vi "Generate Header Vectors.vi"(0 "RFFE RegReadExt Command in":refnum<class "RFFE RegReadExt Command.lvclass">, 11 "error in (no error)":errorcluster) -> (4 "RFFE RegReadExt Command out":refnum<class "RFFE RegReadExt Command.lvclass">, 6 "Header Vectors":string[](array[string]), 15 "error out":errorcluster)   [LabVIEW 2018, in "MIPI RFFE API.lvlib" / "RFFE RegReadExt Command.lvclass"]
uses:
  RFFE RegReadExt Command.lvclass
  Extended Command/RFFE Extended Command.lvclass
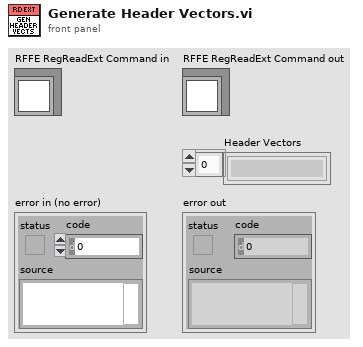
[diagram p1: front panel]
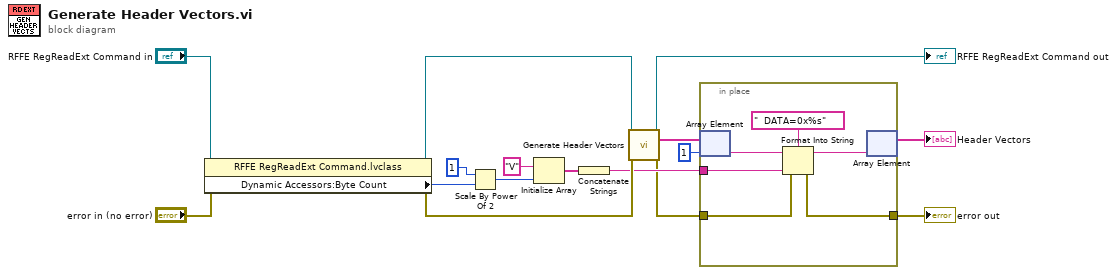
[diagram p0: block diagram]
diagram:
  n1 = property class="RFFE RegReadExt Command.lvclass"(reference="RFFE RegReadExt Command in", error in="error in (no error)") -> (reference out=w14:refnum<class "RFFE RegReadExt Command.lvclass">, error out=w8:errorcluster, "Dynamic Accessors:Byte Count"=w10:i32)
  n2 = Scale By Power Of 2(n=i16 1, x=w10) -> (x*2^n=w6:i32)
  n3 = Initialize Array("V", w6) -> (w4:string[])
  n4 = Concatenate Strings(w4) -> (w3:string)
  n5 = call-parent "Generate Header Vectors.vi"("RFFE Command in"=w14, "error in (no error)"=w8) -> ("RFFE Command out"=→"RFFE RegReadExt Command out":refnum<class "RFFE RegReadExt Command.lvclass">, "Header Vectors"=w12:string[], "error out"=w1:errorcluster)  [unwired: 11 in]
  n6 = in-place {
    in-place-border: w3 -> [w19]
    in-place-border: [w18] -> w2
    in-place-border: w1 -> [w17]
    n7 = in-place-array #1(w12, 1) -> (w22:string)
    n8 = Format Into String(format string="  DATA=0x%s", initial string=w22, error in=w17, w19) -> (resulting string=w21:string, error out=w18:errorcluster)
    n9 = in-place-array #1(w21) -> (→"Header Vectors":string[])  [unwired: 1 out]
  }
  "error out" <- w2
